vi "readData.vi"(8 "error in (no error)":errorcluster, 10 "array":string[][](array[string]), 11 "FileReader in":refnum<class "FileReader.lvclass">) -> (0 "error out":errorcluster, 1 "Array":dbl[][](array[numeric]), 2 "channels":string, 3 "FileReader out":refnum<class "FileReader.lvclass">, 4 "Defaults":dbl[](array[numeric]), 5 "channelAddresses":string[](array[string]))   [LabVIEW 2011, in "Tools.lvlib" / "Filing.lvlib" / "FileReader.lvclass"]
uses:
  FileReader.lvclass
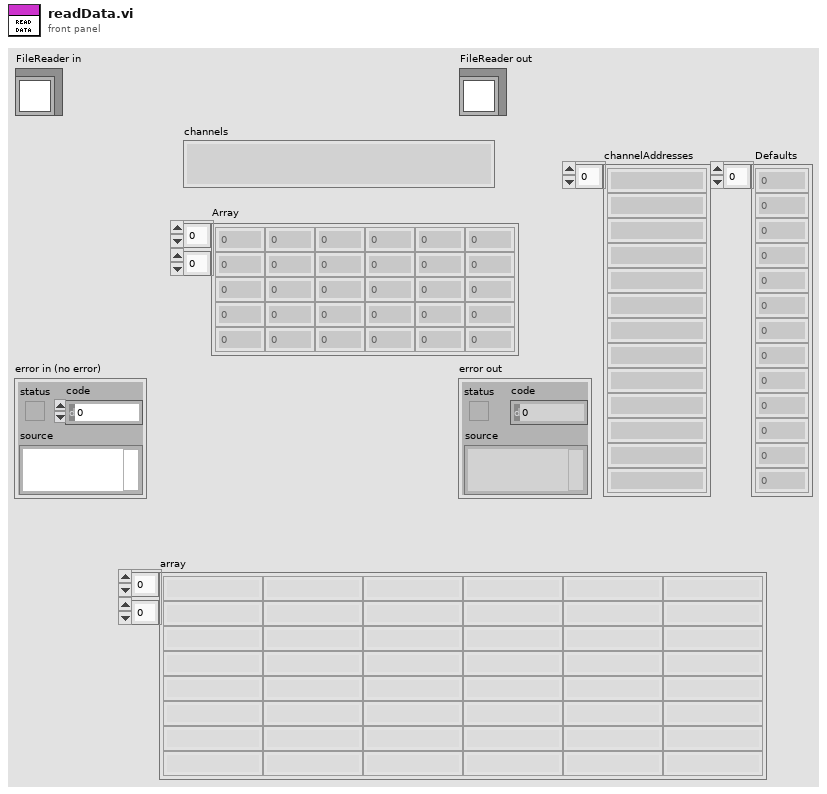
[diagram p1: front panel]
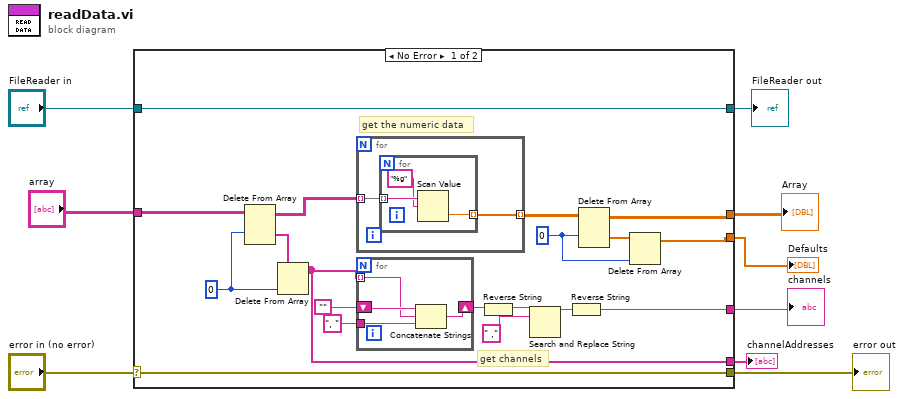
[diagram p0: block diagram]
diagram:
  n1 = case shown="No Error" "error in (no error)" {
    selector: "error in (no error)" -> [w27 w39]
    tunnel: [w27 w39] -> w8
    tunnel: [w28 w38] -> w6
    tunnel: "FileReader in" -> [w28 w38]
    tunnel: "array" -> [w18 _]
    tunnel: [w14 _] -> w4
    tunnel: [w16 _] -> w3
    tunnel: [w11 _] -> w2
    tunnel: [w13 _] -> w1
    frame No Error {
      w10 = 0 ("index (row)")
      w17 = 0 ("index")
      # "get channels"
      # "get the numeric data"
      n2 = Delete From Array(array=w18, index (row)=w17) -> (deleted portion=w21:string[], array with subset deleted=w20:string[][])  [unwired: 2 in]
      n3 = Delete From Array(array=w21, index=w17) -> (array with subset deleted=w13:string[])  [unwired: 1 in, 1 out]
      n4 = for {
        tunnel: w20 -> [w30] mode=indexing
        tunnel: [w29] -> w15 mode=indexing
        n5 = for {
          tunnel: w30 -> [w33] mode=indexing
          tunnel: [w31] -> w29 mode=indexing
          n6 = Scan Value(string=w33, format string="%g") -> (value=w31:dbl)  [unwired: 1 in, 1 out]
        }
      }
      n7 = for {
        tunnel: w13 -> [w36] mode=indexing
        shift-right: [w35] -> w25
        shift-left: "" -> [w37]
        tunnel: ", " -> [w34]
        n8 = Concatenate Strings(w37, w36, w34) -> (w35:string)
      }
      n9 = Reverse String(1:w25) -> (0:w24:string)
      n10 = Search and Replace String(input string=w24, search string=" ,") -> (result string=w22:string)  [unwired: 6 in, 3 out]
      n11 = Reverse String(1:w22) -> (0:w16:string)
      n12 = Delete From Array(array=w15, index (row)=w10) -> (deleted portion=w12:dbl[], array with subset deleted=w14:dbl[][])  [unwired: 2 in]
      n13 = Delete From Array(array=w12, index=w10) -> (array with subset deleted=w11:dbl[])  [unwired: 1 in, 1 out]
    }
    frame Error {
    }
  }
  "error out" <- w8
  "FileReader out" <- w6
  "Array" <- w4
  "channels" <- w3
  "Defaults" <- w2
  "channelAddresses" <- w1
